vi "Insert.vi"(6 "Table Name":string, 8 "error in (no error)":errorcluster, 9 "Data List":variant, 10 "ColumnName List":variant, 11 "DataBase_SQL in":refnum<class "DataBase_SQL.lvclass">) -> (0 "error out":errorcluster, 2 "SQL Query":string, 3 "DataBase_SQL out":refnum<class "DataBase_SQL.lvclass">)   [LabVIEW 2021, in "DataBase_SQL.lvclass"]
uses:
  <userlib>/John_Lib/DataBase/DataBase_SQL/DataBase_SQL.lvclass
  <userlib>/John_Lib/DataBase/DataBase_SQL/DataBase_SQL.lvclass/DataBase_SQL.ctl
  cc901b8c-21a1-430b-99f2-dd2fbbcd1733.vi
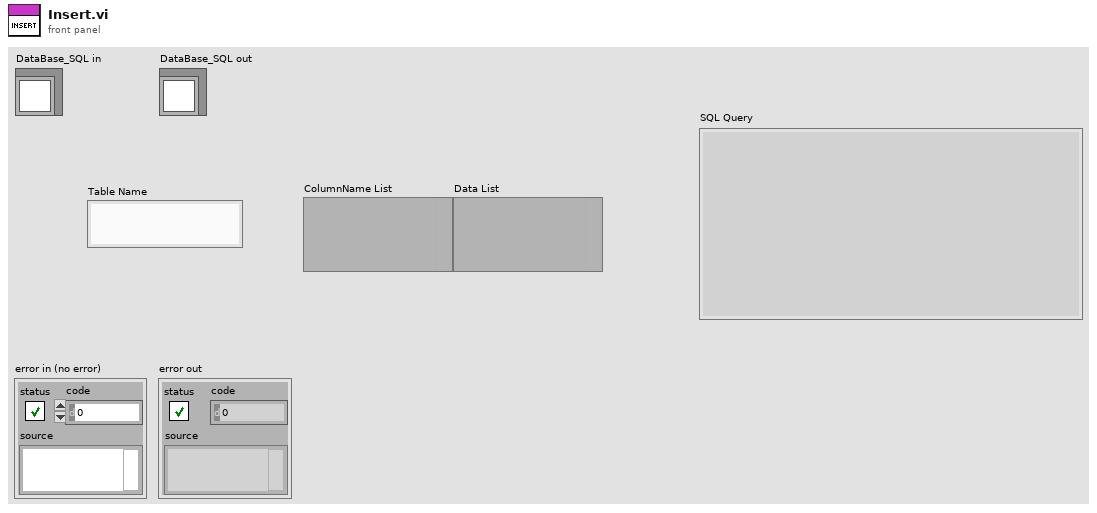
[diagram p1: front panel]
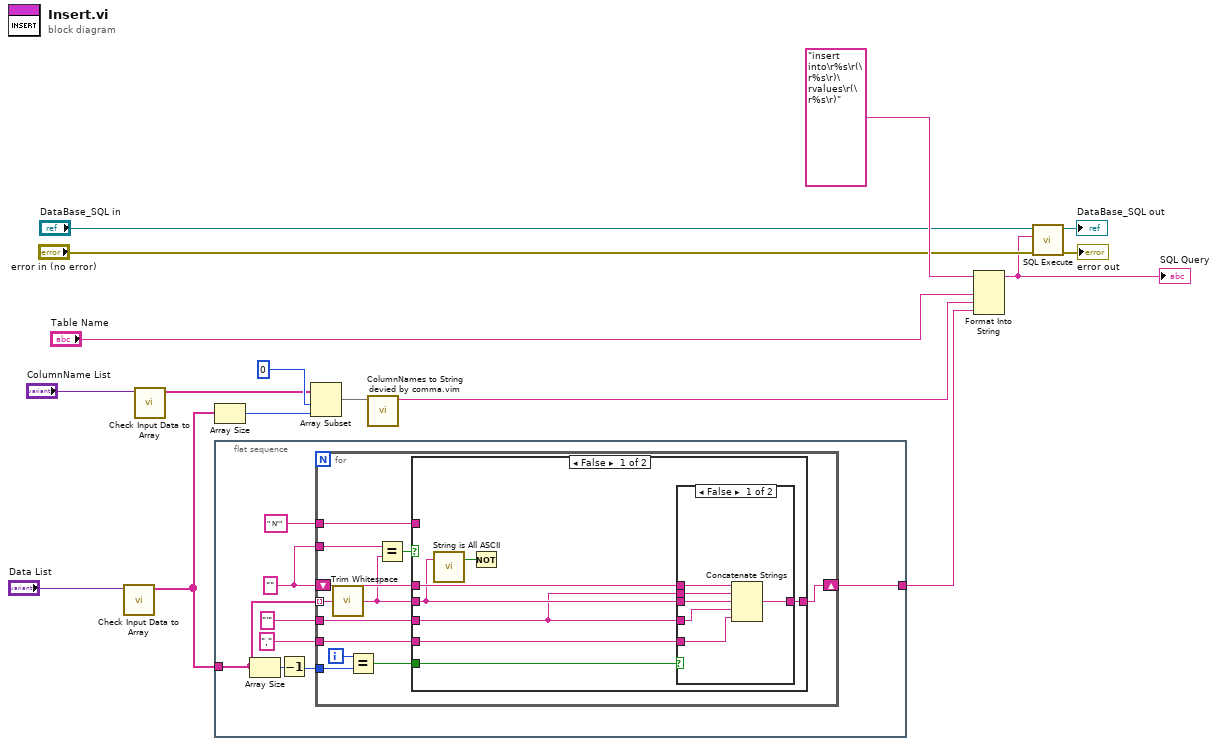
[diagram p0: block diagram]
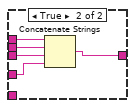
[diagram p2: hidden frame]
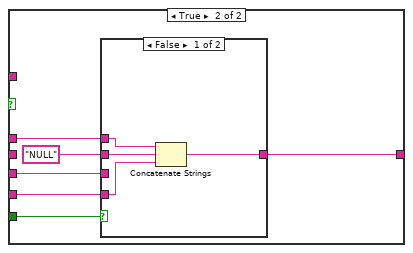
[diagram p3: hidden frame]
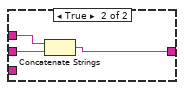
[diagram p4: hidden frame]
diagram:
  n1 = call <userlib>:"Check Input Data to Array.vi"("String Array/ String"="Data List") -> ("ColumnsNameList"=w1:string[])  [unwired: 9 in, 1 out]
  n2 = call <userlib>:"Check Input Data to Array.vi"("String Array/ String"="ColumnName List") -> ("ColumnsNameList"=w3:string[])  [unwired: 9 in, 1 out]
  n3 = Array Size(array=w1) -> (size(s)=w11:i32)
  n4 = flat-sequence {
    tunnel: w1 -> [w18]
    tunnel: [w17] -> w16
    frame #0 {
      w23 = "" ("string")
      n5 = Array Size(array=w18) -> (size(s)=w21:i32)
      n6 = Decrement(x=w21) -> (x-1=w22:i32)
      n7 = for {
        tunnel: w18 -> [w29] mode=indexing
        shift-right: [w30] -> w17
        shift-left: w23 -> [w31]
        tunnel: "'" ("string") -> [w36]
        tunnel: "," ("string") -> [w35]
        tunnel: w22 -> [w33]
        tunnel: w23 -> [w28]
        tunnel: " N'" ("string") -> [w26]
        i -> [w34]
        n8 = call <vilib>:"Trim Whitespace.vi"("string"=w29) -> ("trimmed string"=w25:string)  [unwired: 1 in]
        n9 = Equal?(x=w34, y=w33) -> (x = y?=w32:bool)
        n10 = Equal?(x=w28, y=w25) -> (x = y?=w27:bool)
        n11 = case shown="False" w27 {
          tunnel: w25 -> [w39 _]
          tunnel: w36 -> [w37 w60]
          tunnel: w35 -> [w43 w59]
          tunnel: w32 -> [w42 w58]
          tunnel: w31 -> [w41 w57]
          tunnel: [w40 w56] -> w30
          tunnel: w26 -> [_ _]
          frame False {
            n12 = call <userlib>:"String is All ASCII.vi"("string In"=w39) -> ("All is ASCII？"=w38:bool)  [unwired: 2 in]
            n13 = Not(x=w38) -> ()  [unwired: 1 out]
            n14 = case shown="False" w42 {
              tunnel: w39 -> [w49 w54]
              tunnel: [w48 w53] -> w40
              tunnel: w37 -> [w47 w52]
              tunnel: w43 -> [w46 _]
              tunnel: w41 -> [w45 w51]
              tunnel: w37 -> [w44 w50]
              frame False {
                n15 = Concatenate Strings(w45, w44, w49, w47, w46) -> (w48:string)
              }
              frame True {
                n16 = Concatenate Strings(w51, w50, w54, w52) -> (w53:string)
              }
            }
          }
          frame True {
            # "NULL 的两旁没有单引号。\n2014-11-13 14:18:33"
            n17 = case shown="False" w58 {
              tunnel: "NULL" ("Double all the singe quotation Mark in the string") -> [w64 w67]
              tunnel: [w63 w66] -> w56
              tunnel: w60 -> [_ _]
              tunnel: w59 -> [w62 _]
              tunnel: w57 -> [w61 w65]
              frame False {
                n18 = Concatenate Strings(w61, w64, w62) -> (w63:string)
              }
              frame True {
                n19 = Concatenate Strings(w65, w67) -> (w66:string)
              }
            }
          }
        }
      }
    }
  }
  n20 = Array Subset(array=w3, index=0, length=w11) -> (w13:string[])
  n21 = call "ColumnNames to String devied by comma.vim"("ColumnNames"=w13) -> ("Columns,String"=w15:string)  [unwired: 10 in]
  n22 = Format Into String(format string="insert into\r%s\r(\r%s\r)\rvalues\r(\r%s\r)", "Table Name", w15, w16) -> (resulting string=w5:string)  [unwired: 2 in, 1 out]
  "SQL Query" <- w5
  n23 = call-dynamic "SQL Execute.vi"("error in (no error)"="error in (no error)", "Command Text"=w5, "DataBase_SQL in"="DataBase_SQL in") -> ("error out"=→"error out":errorcluster, "DataBase_SQL out"=→"DataBase_SQL out":refnum<class "DataBase_SQL.lvclass">)  [unwired: 4 in, 3 out]
